vi "lvssh2_session_callback_register_kbdint_response_64.vi"(11 "keyboard-interactive response":refnum<vi>) -> (0 "error out":errorcluster, 2 "stop event":refnum<user-event>, 3 "user event":refnum<user-event>)   [LabVIEW 2017, in "libssh2.lvlib"]
uses:
  libssh2.lvlib
  lvssh2_userauth_keyboard_interactive_response_function_input_args_64.ctl
  lvssh2_userauth_keyboard_interactive_response_function_handler_64.vi
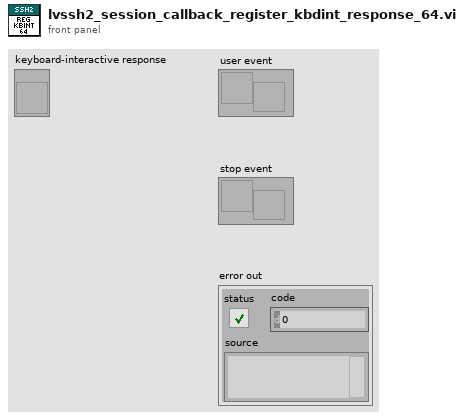
[diagram p1: front panel]
types:
  T1 = typedef "libssh2.lvlib/lvssh2_userauth_keyboard_interactive_response_function_input_args_64.ctl" = cluster{"name":string, "instruction":string, "num_prompts":i32, "*prompts":u64, "*responses":u64, "completion":u64}
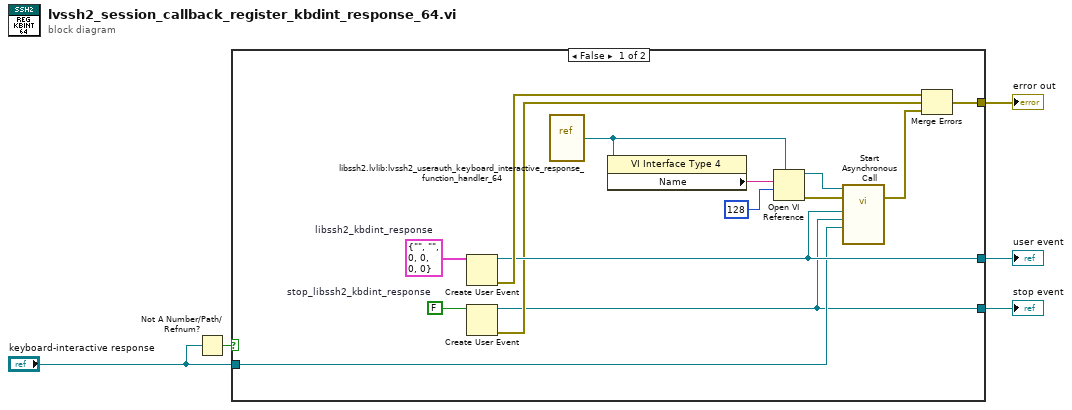
[diagram p0: block diagram]
diagram:
  n1 = Not A Number/Path/Refnum?(number/path/refnum="keyboard-interactive response") -> (NaN/Path/Refnum?=w3:bool)
  n2 = case shown="False" w3 {
    tunnel: [w10 _] -> w5
    tunnel: [w6 _] -> w1
    tunnel: [w19 _] -> w4
    tunnel: "keyboard-interactive response" -> [w9 _]
    frame False {
      w8 = FALSE  # stop_libssh2_kbdint_response
      w18 = T1 {"name"="", "instruction"="", "num_prompts"=0, "*prompts"=0, "*responses"=0, "completion"=0}  # libssh2_kbdint_response
      n3 = Create User Event(user event datatype=w18) -> (user event=w10:refnum<user-event>, error out=w17:errorcluster)  [unwired: 1 in]
      n4 = Create User Event(user event datatype=w8) -> (user event=w6:refnum<user-event>, error out=w7:errorcluster)  [unwired: 1 in]
      n5 = vi-ref "libssh2.lvlib:lvssh2_userauth_keyboard_interactive_response_function_handler_64.vi"() -> ("vi reference"=w16:refnum<vi>)
      n6 = property class="VI Interface Type 4"(reference=w16) -> ("Name"=w15:string)  [unwired: 1 in, 2 out]
      n7 = Open VI Reference(type specifier VI Refnum (for type only)=w16, vi path=w15, options=128) -> (vi reference=w11:refnum<vi>, error out=w12:errorcluster)  [unwired: 3 in]
      n8 = call-by-ref "Start Asynchronous Call"(reference=w11, error in=w12, "lvssh2_userauth_keyboard_interactive_response_function"=w9, "Stop Event Ref"=w6, "User Event Ref"=w10) -> (error out=w13:errorcluster)  [unwired: 9 in, 1 out]
      n9 = Merge Errors(w17, w7, w13) -> (w19:errorcluster)
    }
    frame True {
    }
  }
  "user event" <- w5
  "error out" <- w4
  "stop event" <- w1
